vi "EVAL-AD5764EB Write.vi"(8 "error in (no error)":errorcluster, 9 "Voltage":dbl, 10 "Chanel":u16(ring) items=["A", "B", "C", "D"], 11 "VISA resource name":refnum<visa-resource-name>) -> (0 "error out":errorcluster, 3 "VISA resource name out":refnum<visa-resource-name>)   [LabVIEW 2018, in "EVAL-AD5764EB.lvlib"]
uses:
  EVAL-AD5764EB.lvlib
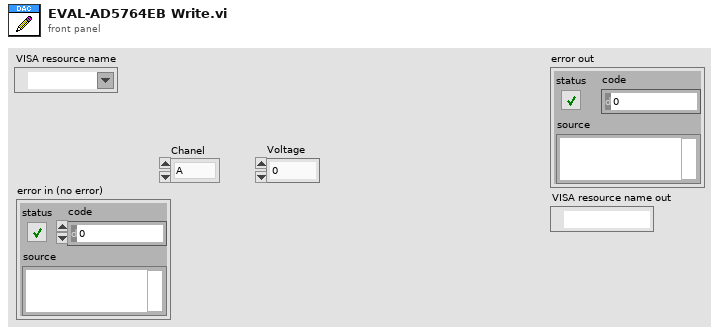
[diagram p1: front panel]
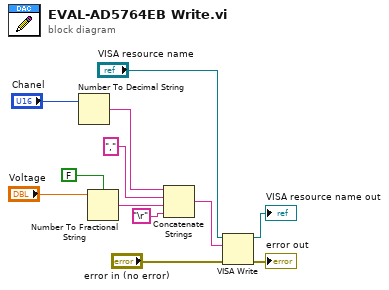
[diagram p0: block diagram]
diagram:
  n1 = Number To Decimal String(number="Chanel") -> (decimal integer string=w6:string)  [unwired: 1 in]
  n2 = Number To Fractional String(use system decimal point (T)=FALSE, number="Voltage") -> (F-format string=w5:string)  [unwired: 2 in]
  n3 = Concatenate Strings(w6, ",", w5, "\r") -> (w2:string)
  n4 = VISA Write(VISA resource name="VISA resource name", write buffer=w2, error in (no error)="error in (no error)") -> (VISA resource name out=→"VISA resource name out":refnum<visa-resource-name>, error out=→"error out":errorcluster)  [unwired: 1 out]
